vi "Extract_to_TSV.vi"() -> ()   [LabVIEW 2019]
panel:
  in  "Output file name":string
  in  "OK":bool
  in  "Samples to average":i32=10000
  in  "Samples per freq calc":i32=10000
  in  "Folder":path
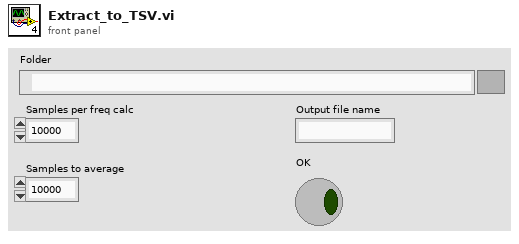
[diagram p1: front panel]
types:
  T1 = enum16{"open", "replace", "create", "open or create", "replace or create", "replace or create with confirmation"}
  T2 = enum16{"open", "open or create", "create or replace", "create", "open (read-only)"}
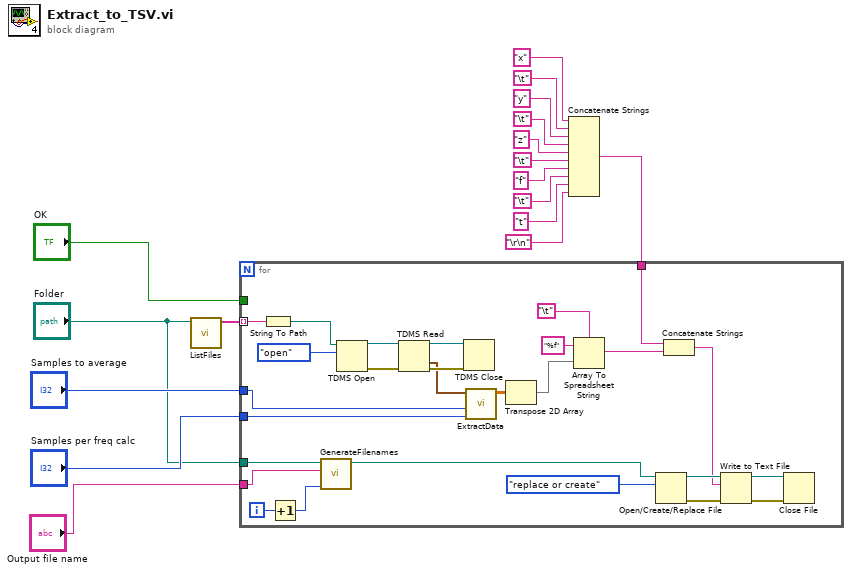
[diagram p0: block diagram]
diagram:
  n1 = call "ListFiles.vi"("Folder"="Folder") -> ("TDMS"=w16:string[])  [unwired: 10 in]
  n2 = Concatenate Strings("x" ("string"), "\t", "y" ("string"), "\t", "z" ("string"), "\t", "f" ("string"), "\t", "t" ("string"), "\r\n") -> (w10:string)
  n3 = for {
    tunnel: "Samples per freq calc" -> [w38]
    tunnel: w16 -> [w32] mode=indexing
    tunnel: "Samples to average" -> [w31]
    tunnel: "OK" -> [_]
    tunnel: "Folder" -> [w25]
    tunnel: "Output file name" -> [w22]
    tunnel: w10 -> [w19]
    i -> [w24]
    n4 = String To Path(string=w32) -> (path=w30:path)
    n5 = Increment(x=w24) -> (x+1=w23:i32)
    n6 = call "GenerateFilenames.vi"("file number"=w23, "filename"=w22, "Path"=w25) -> ("Filepath"=w21:path)  [unwired: 8 in]
    n7 = TDMS Open(10:T2."open" ("operation (0:open)"), 11:w30) -> (0:w42:errorcluster, 3:w43:refnum<k34>)  [unwired: 5 in]
    n8 = TDMS Read(0:w43, 11:w42) -> (4:w41:refnum<k34>, 10:w39:waveform(dbl)[], 15:w40:errorcluster)  [unwired: 6 in, 3 out]
    n9 = TDMS Close(8:w40, 11:w41) -> ()  [unwired: 2 out]
    n10 = call "ExtractData.vi"("Samples per freq calc"=w38, "Samples to average"=w31, "Data input"=w39) -> ("Data array"=w29:dbl[][])  [unwired: 8 in]
    n11 = Transpose 2D Array(2D array=w29) -> (transposed array=w27:dbl[][])
    n12 = Array To Spreadsheet String(delimiter (Tab)="\t", array=w27, 3:"%f" ("format string")) -> (spreadsheet string=w18:string)
    n13 = Open/Create/Replace File(file path (use dialog)=w21, operation (0:open)=T1."replace or create") -> (refnum out=w35:refnum<file>, error out=w34:errorcluster)  [unwired: 4 in, 1 out]
    n14 = Concatenate Strings(w19, w18) -> (w20:string)
    n15 = Write to Text File(file (use dialog)=w35, text=w20, error in=w34) -> (refnum out=w37:refnum<file>, error out=w36:errorcluster)  [unwired: 1 in, 1 out]
    n16 = Close File(refnum=w37, error in=w36) -> ()  [unwired: 2 out]
  }
